vi "Renishaw-XL80_SetSlowAveraging.vi"(8 "error in (no error)":errorcluster, 11 "Renishaw-XL80 in":refnum<class "Renishaw-XL80.lvclass">) -> (0 "error out":errorcluster, 3 "Renishaw-XL80 out":refnum<class "Renishaw-XL80.lvclass">)   [LabVIEW 2024, in "Renishaw-XL80.lvclass"]
doc: "This method will set long-term averaging of the ML10 count on.\n\nDefinition\nHRESULTSetSlowAveraging();\nParameters\nNone\n\nComments\nThis method will return with an HRESULT of E_FAIL if the client has not previously connected to a DX10 by calling Connect. The method will also return E_FAIL if the DX10 is not responding or the ML10 is not responding.Otherwise the method will return an HRESULT of S_OK.\n\nLong term (slow) averaging enables a \"box car\" averaging algorithm inside the ML10 with a response time of approximately 4secs.\n\nNote that short term averaging is on when the ML10 status has both ML10_AVERAGING_ON and ML10_LONG_TERM_AVERAGING_ON set.\n\nNote that averaging has no effect on synchronous TPin triggered readings."
uses:
  Renishaw-XL80.lvclass
  Renishaw-XL80.lvclass/Renishaw-XL80.ctl
  D:/A.C.M/Example CSharp_64/bin/Debug/Interop.DX10SDKADAPTORLib.dll
  Example CSharp_64/bin/Debug/Interop.DX10SDKADAPTORLib.dll
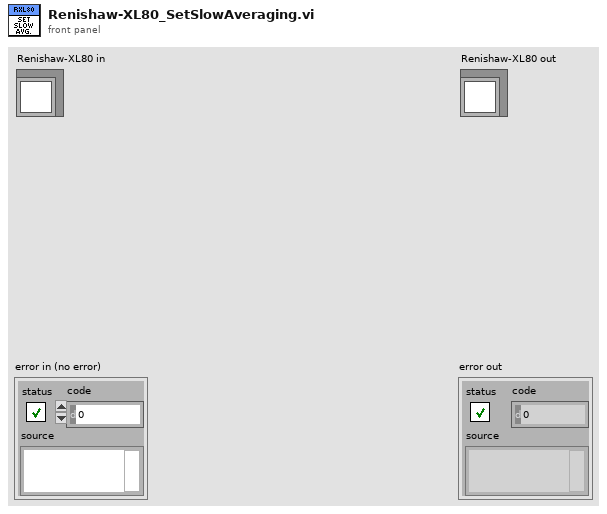
[diagram p1: front panel]
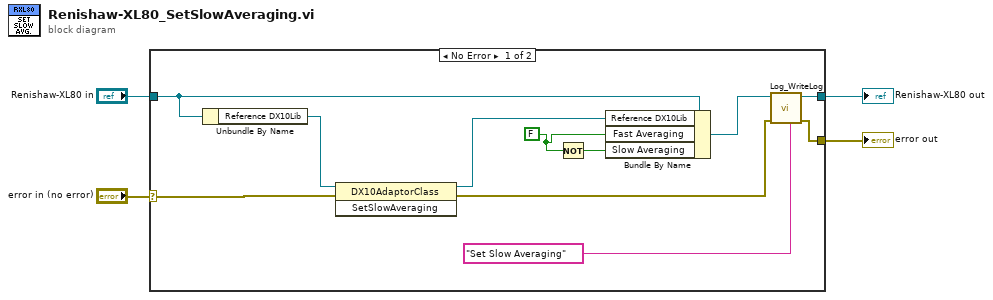
[diagram p0: block diagram]
diagram:
  n1 = case shown="No Error" "error in (no error)" {
    selector: "error in (no error)" -> [w10 w17]
    tunnel: [w9 w17] -> w3
    tunnel: [w8 w16] -> w1
    tunnel: "Renishaw-XL80 in" -> [w7 w16]
    frame No Error {
      w6 = FALSE ("Fast Averaging")
      n2 = Unbundle By Name(w7) -> ("Reference DX10Lib"=w11:refnum<k24>)
      n3 = invoke class="DX10AdaptorClass" method="SetSlowAveraging"(reference=w11, error in=w10) -> (reference out=w13:refnum<k24>, error out=w14:errorcluster)  [unwired: 1 in, 1 out]
      n4 = Not(x=w6) -> (.not. x?=w5:bool)
      n5 = Bundle By Name(cluster=w7, "Reference DX10Lib"=w13, "Fast Averaging"=w6, "Slow Averaging"=w5) -> (w12:refnum<class "Renishaw-XL80.lvclass">)
      n6 = call-dynamic "Log_WriteLog.vi"("Additional text"="Set Slow Averaging", "error in (no error)"=w14, "Log in"=w12) -> ("error out"=w9:errorcluster, "Log out"=w8:refnum<class "Renishaw-XL80.lvclass">)  [unwired: 7 in]
    }
    frame Error {
    }
  }
  "error out" <- w3
  "Renishaw-XL80 out" <- w1
